vi "LUT_CharsetBlue.vi"() -> (0 "Init Data Out":bool[](array[boolean]))   [LabVIEW 2018]
panel:
  # "For Initialization VI requirements and help, please read directions located on Block Diagram."
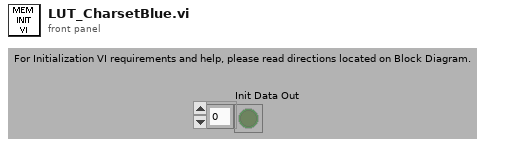
[diagram p1: front panel]
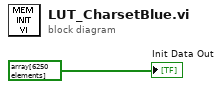
[diagram p0: block diagram]
diagram:
  "Init Data Out" <- bool[] array[6250 elements] ("Blue_LUT")
